vi "Test-SharedVariable2.vi"() -> ()   [LabVIEW 2014]
panel:
  out "error IO":errorcluster
  out "读取共享变量":i32(listbox)
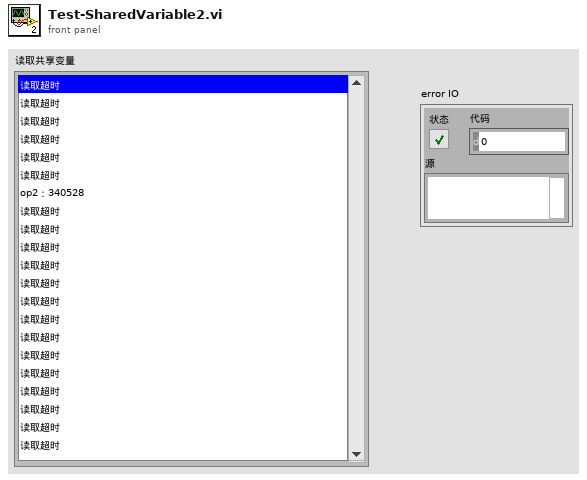
[diagram p1: front panel]
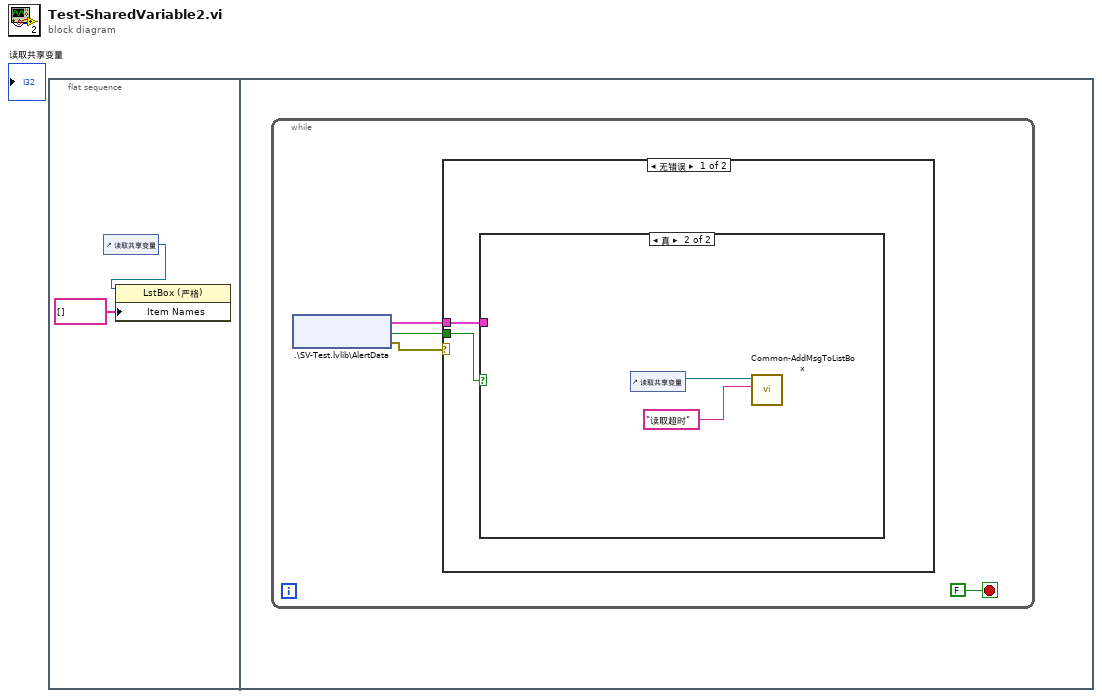
[diagram p0: block diagram]
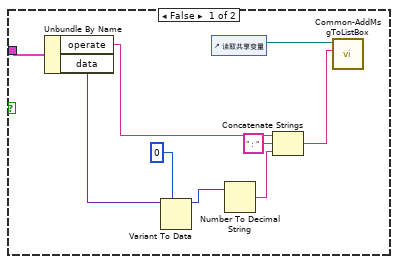
[diagram p2: hidden frame]
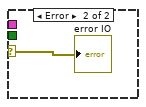
[diagram p3: hidden frame]
diagram:
  n1 = flat-sequence {
    frame #0 {
      n2 = control-ref of="读取共享变量"() -> (w1:refnum<vi>)
      n3 = property class="LstBox (严格)"(reference=w1, "Item Names"=string[] [] ("项名")) -> ()  [unwired: 1 in, 2 out]
    }
    frame #1 {
      n4 = while {
        stop <- FALSE stop-if-true
        n5 = shared-variable ".\\SV-Test.lvlib\\AlertData"() -> (w6:cluster{"operate":string, "data":variant}, error out=w4:errorcluster, w3:bool)  [unwired: 2 in]
        n6 = case shown="无错误" w4 {
          selector: w4 -> [_ w20]
          tunnel: w6 -> [w8 _]
          tunnel: w3 -> [w7 _]
          frame No Error {
            n7 = case shown="真" w7 {
              tunnel: w8 -> [w17 _]
              frame False {
                n8 = Unbundle By Name(w17) -> ("operate"=w15:string, "data"=w13:variant)
                n9 = Variant To Data(type=0, Variant=w13) -> (data=w11:i32)  [unwired: 1 in, 1 out]
                n10 = control-ref of="读取共享变量"() -> (w16:refnum<vi>)
                n11 = Number To Decimal String(number=w11) -> (decimal integer string=w10:string)  [unwired: 1 in]
                n12 = Concatenate Strings(w15, "：" ("字符串"), w10) -> (w9:string)
                n13 = call "Common-AddMsgToListBox.vi"("字符串"=w9, "列表框"=w16) -> ()  [unwired: 10 in]
              }
              frame True {
                n14 = control-ref of="读取共享变量"() -> (w19:refnum<vi>)
                n15 = call "Common-AddMsgToListBox.vi"("字符串"="读取超时", "列表框"=w19) -> ()  [unwired: 10 in]
              }
            }
          }
          frame Error {
            "error IO" <- w20
          }
        }
      }
    }
  }
